vi "WriteMaxDataInputSize.vi"(8 "Error In":errorcluster, 9 "Max Data Input Size":i32=-1) -> (0 "Error Out":errorcluster)   [LabVIEW 2018, in "TracerLibrary.lvlib" / "Tracer.lvclass"]
uses:
  Tracer.lvclass
  protected/Tracer_ClassAttributes.vi
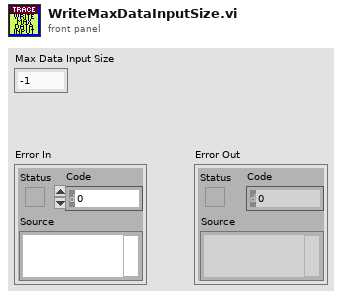
[diagram p1: front panel]
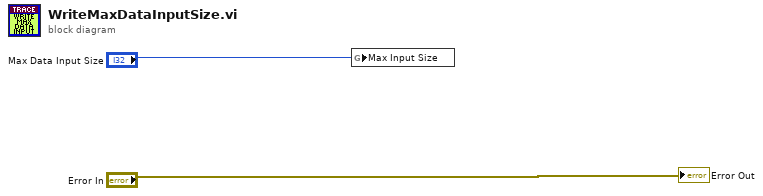
[diagram p0: block diagram]
diagram:
  n1 = global write "Tracer_ClassAttributes.vi" "Max Input Size"("Max Data Input Size") -> ()
  "Error Out" <- "Error In"
